vi "front-panel.vi"   [LabVIEW 2026]
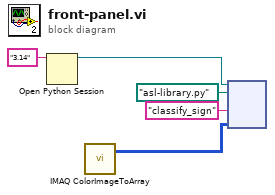
[diagram p0: block diagram]
diagram:
  n1 = Open Python Session(python version="3.14" ("Python version")) -> (session out=w2:refnum<k35>)  [unwired: 2 in, 1 out]
  n2 = call "IMAQ ColorImageToArray"() -> ("Image Pixels (U32)"=w1:u32[][])  [unwired: 4 in, 2 out]
  n3 = node(w2, path "asl-library.py" ("module path"), "classify_sign" ("function name"), w1) -> ()  [unwired: 4 in, 4 out]
